vi "Replace String Tokens.vi"(10 "String":string) -> (2 "String out":string)   [LabVIEW 2016, in "CLD Exam - ATM.lvlib" / "Terminal Message.lvclass"]
uses:
  Terminal Message.lvclass
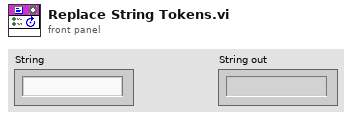
[diagram p1: front panel]
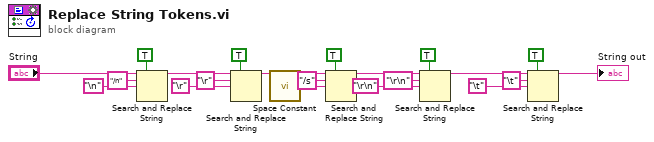
[diagram p0: block diagram]
diagram:
  n1 = Search and Replace String(replace all?=TRUE ("replace all? (F)"), input string="String", search string="/n", replace string="\n") -> (result string=w16:string)  [unwired: 4 in, 3 out]
  n2 = Search and Replace String(replace all?=TRUE ("replace all? (F)"), input string=w16, search string="\r" ("String 2"), replace string="\r") -> (result string=w6:string)  [unwired: 4 in, 3 out]
  n3 = call <vilib>:"Space Constant.vi"() -> ("String"=w9:string)
  n4 = Search and Replace String(replace all?=TRUE ("replace all? (F)"), input string=w6, search string="/s", replace string=w9) -> (result string=w11:string)  [unwired: 4 in, 3 out]
  n5 = Search and Replace String(replace all?=TRUE ("replace all? (F)"), input string=w11, search string="\r\n" ("String 2"), replace string="\r\n") -> (result string=w2:string)  [unwired: 4 in, 3 out]
  n6 = Search and Replace String(replace all?=TRUE ("replace all? (F)"), input string=w2, search string="\t" ("String 2"), replace string="\t") -> (result string=→"String out":string)  [unwired: 4 in, 3 out]
